vi "lia_fpga_array.vi"() -> ()   [LabVIEW 2009]
uses:
  <vilib>/eio/EIONode/EIONode.xnode
  <vilib>/rvi/eio/nirviEIOImplementation/nirviEIOImplementation.xnode
  <vilib>/rvi/eio/common/nirviEmuTemplateMethod_noerrors.vi
  <vilib>/rvi/eio/common/nirviEmuClasses.ctl
panel:
  out "XY_fpga":i32[](array[numeric])
  in  "beta":i32[](array[numeric])=[0, 0, 0, 0, 0, 0]
  in  "Signal Amplitude 3":u16
  in  "Phase Shift 3":u32
  in  "Accumulator Increment 3":u32
  in  "Signal Amplitude 2":u16
  in  "Phase Shift 2":u32
  in  "Accumulator Increment 2":u32
  in  "stop":bool
  out "Actual Gen Rate (ticks)":u32
  in  "Update Rate (ticks)":u32
  in  "Signal Amplitude 1":u16
  in  "Phase Shift 1":u32
  in  "Accumulator Increment 1":u32
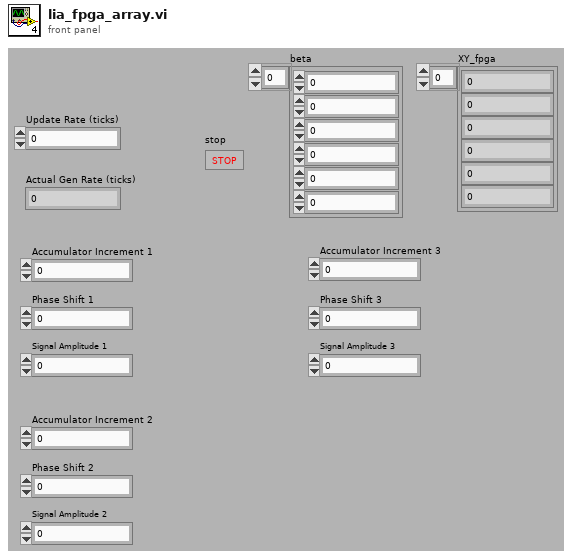
[diagram p1: front panel]
types:
  T1 = typedef "nirviEmuClasses.ctl" = enum16{"IO Read", "IO Write", "Method", "Property Read", "Property Write"}
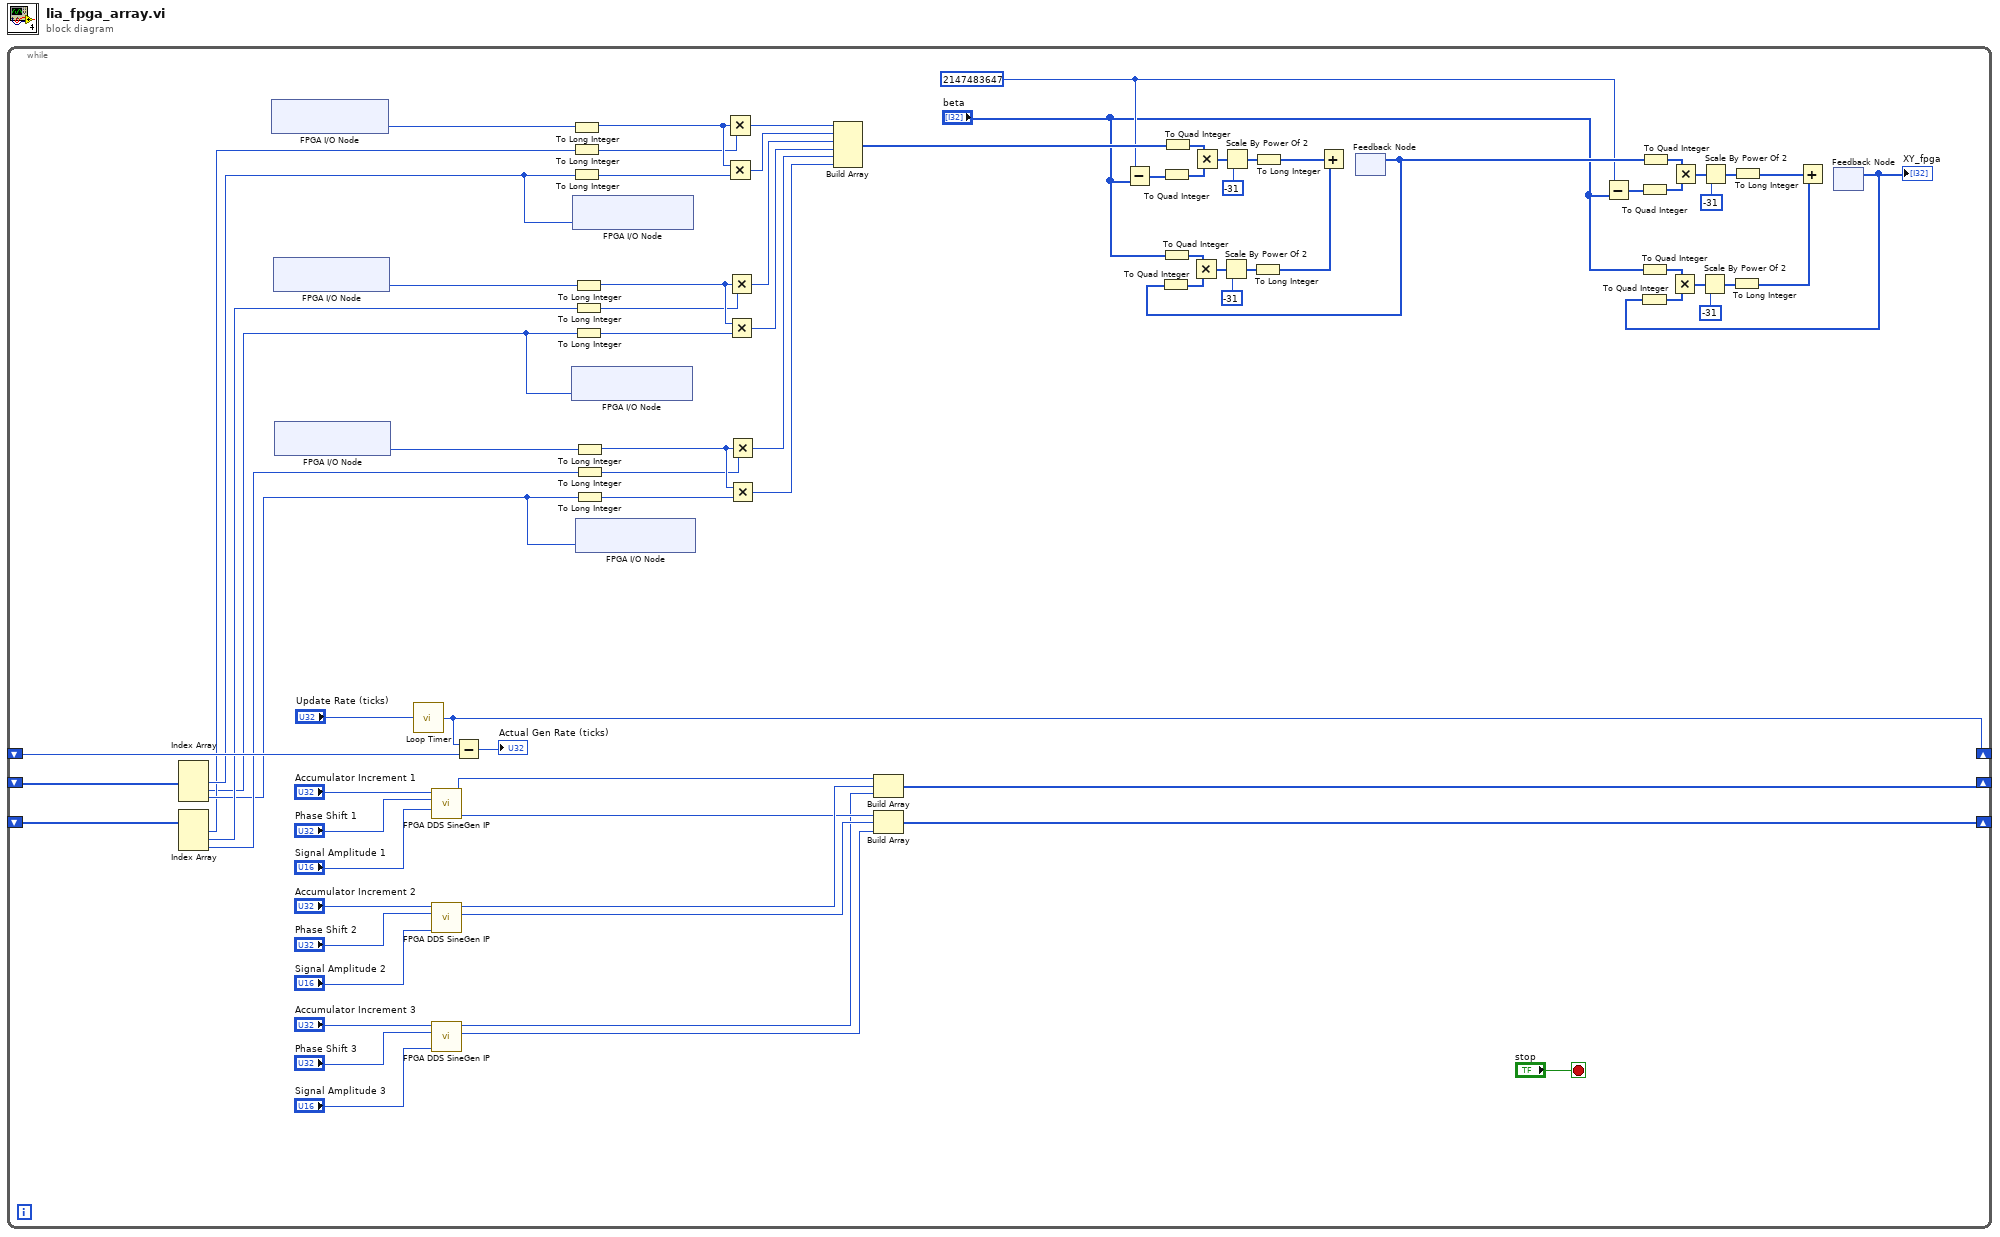
[diagram p0: block diagram]
diagram:
  n1 = while {
    shift-right: [w61] -> _
    shift-left: _ -> [w59]
    shift-right: [w78] -> _
    shift-left: _ -> [w76]
    shift-right: [w60] -> _
    shift-left: _ -> [w57]
    stop <- "stop" stop-if-true
    w3 = 2147483647
    n2 = Index Array(array=w59) -> (element #1=w58:i16, element #2=w19:i16, element #3=w41:i16)  [unwired: 3 in]
    n3 = Index Array(array=w57) -> (element #1=w20:i16, element #2=w52:i16, element #3=w42:i16)  [unwired: 3 in]
    n4 = xnode "FPGA I/O Node"() -> ("Connector0/AI0"=w72:i16)  [unwired: 1 in, 1 out]
    n5 = xnode "FPGA I/O Node"() -> ("Connector0/AI1"=w56:i16)  [unwired: 1 in, 1 out]
    n6 = xnode "FPGA I/O Node"() -> ("Connector0/AI2"=w46:i16)  [unwired: 1 in, 1 out]
    n7 = call "Loop Timer"("Count(Ticks)"="Update Rate (ticks)") -> ("Tick Count(Ticks)"=w78:u32)
    n8 = call "FPGA DDS SineGen IP.vi"("Signal Amplitude (x 2^15)"="Signal Amplitude 1", "Phase Shift"="Phase Shift 1", "Accumulator Increment"="Accumulator Increment 1") -> ("Cos output"=w63:i16, "Sin output"=w65:i16)  [unwired: 6 in, 1 out]
    n9 = call "FPGA DDS SineGen IP.vi"("Signal Amplitude (x 2^15)"="Signal Amplitude 2", "Phase Shift"="Phase Shift 2", "Accumulator Increment"="Accumulator Increment 2") -> ("Cos output"=w62:i16, "Sin output"=w64:i16)  [unwired: 6 in, 1 out]
    n10 = call "FPGA DDS SineGen IP.vi"("Signal Amplitude (x 2^15)"="Signal Amplitude 3", "Phase Shift"="Phase Shift 3", "Accumulator Increment"="Accumulator Increment 3") -> ("Cos output"=w47:i16, "Sin output"=w48:i16)  [unwired: 6 in, 1 out]
    n11 = Subtract(x=w78, y=w76) -> (x-y=→"Actual Gen Rate (ticks)":u32)
    n12 = To Long Integer(number=w72) -> (32bit integer=w71:i32)
    n13 = To Long Integer(number=w20) -> (32bit integer=w70:i32)
    n14 = To Long Integer(number=w58) -> (32bit integer=w69:i32)
    n15 = xnode "FPGA I/O Node"("Connector0/AO1"=w19) -> ()  [unwired: 1 in, 1 out]
    n16 = xnode "FPGA I/O Node"("Connector0/AO0"=w58) -> ()  [unwired: 1 in, 1 out]
    n17 = To Long Integer(number=w56) -> (32bit integer=w55:i32)
    n18 = To Long Integer(number=w52) -> (32bit integer=w54:i32)
    n19 = To Long Integer(number=w19) -> (32bit integer=w53:i32)
    n20 = To Long Integer(number=w46) -> (32bit integer=w45:i32)
    n21 = To Long Integer(number=w42) -> (32bit integer=w44:i32)
    n22 = To Long Integer(number=w41) -> (32bit integer=w43:i32)
    n23 = xnode "FPGA I/O Node"("Connector0/AO2"=w41) -> ()  [unwired: 1 in, 1 out]
    n24 = Multiply(x=w71, y=w70) -> (x*y=w27:i32)
    n25 = Multiply(x=w71, y=w69) -> (x*y=w26:i32)
    n26 = Multiply(x=w55, y=w54) -> (x*y=w25:i32)
    n27 = Multiply(x=w55, y=w53) -> (x*y=w24:i32)
    n28 = Multiply(x=w45, y=w44) -> (x*y=w23:i32)
    n29 = Multiply(x=w45, y=w43) -> (x*y=w22:i32)
    n30 = Build Array(w27, w26, w25, w24, w23, w22) -> (w21:i32[])
    n31 = Build Array(w65, w64, w48) -> (w61:i16[])
    n32 = Build Array(w63, w62, w47) -> (w60:i16[])
    n33 = Subtract(x=w3, y="beta") -> (x-y=w37:i32[])
    n34 = To Quad Integer(1:w37) -> (0:w35:i64[])
    n35 = To Quad Integer(1:"beta") -> (0:w30:i64[])
    n36 = To Quad Integer(1:w21) -> (0:w36:i64[])
    n37 = Multiply(x=w36, y=w35) -> (x*y=w40:i64[])
    n38 = Scale By Power Of 2(n=i16 -31, x=w40) -> (x*2^n=w38:i64[])
    n39 = To Long Integer(number=w38) -> (32bit integer=w34:i32[])
    n40 = feedback #1() -> (w4:i32[])  [unwired: 1 in]
    n41 = To Quad Integer(1:w4) -> (0:w29:i64[])
    n42 = Multiply(x=w30, y=w29) -> (x*y=w33:i64[])
    n43 = Scale By Power Of 2(n=i16 -31, x=w33) -> (x*2^n=w31:i64[])
    n44 = To Long Integer(number=w31) -> (32bit integer=w28:i32[])
    n45 = Add(x=w34, y=w28) -> (x+y=w73:i32[])
    n46 = Subtract(x=w3, y="beta") -> (x-y=w14:i32[])
    n47 = To Quad Integer(1:w14) -> (0:w12:i64[])
    n48 = To Quad Integer(1:"beta") -> (0:w7:i64[])
    n49 = To Quad Integer(1:w4) -> (0:w13:i64[])
    n50 = Multiply(x=w13, y=w12) -> (x*y=w17:i64[])
    n51 = Scale By Power Of 2(n=i16 -31, x=w17) -> (x*2^n=w15:i64[])
    n52 = To Long Integer(number=w15) -> (32bit integer=w11:i32[])
    n53 = feedback #2() -> (w1:i32[])  [unwired: 1 in]
    "XY_fpga" <- w1
    n54 = To Quad Integer(1:w1) -> (0:w6:i64[])
    n55 = Multiply(x=w7, y=w6) -> (x*y=w10:i64[])
    n56 = Scale By Power Of 2(n=i16 -31, x=w10) -> (x*2^n=w8:i64[])
    n57 = To Long Integer(number=w8) -> (32bit integer=w5:i32[])
    n58 = Add(x=w11, y=w5) -> (x+y=w18:i32[])
  }
